vi "copyFuncArgAndNoteFromIniToTable.vi"(8 "valInCol5":string, 9 "valInCol2":string, 10 "valInCol1":string, 11 "arrayAtTheSameRow":string[](array[string])) -> (3 "arrWithFunc&Arg&Note":string[](array[string]))   [LabVIEW 2010]
panel:
  # "func"
  # "arg"
  # "note"
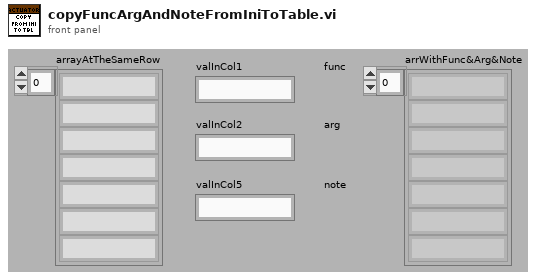
[diagram p1: front panel]
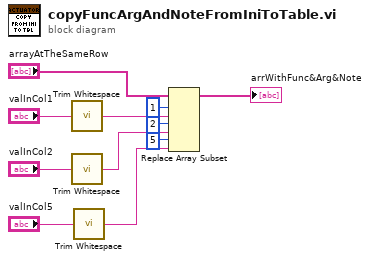
[diagram p0: block diagram]
diagram:
  n1 = call <vilib>:"Trim Whitespace.vi"("string"="valInCol1") -> ("trimmed string"=w5:string)  [unwired: 1 in]
  n2 = call <vilib>:"Trim Whitespace.vi"("string"="valInCol2") -> ("trimmed string"=w4:string)  [unwired: 1 in]
  n3 = call <vilib>:"Trim Whitespace.vi"("string"="valInCol5") -> ("trimmed string"=w3:string)  [unwired: 1 in]
  n4 = Replace Array Subset(array="arrayAtTheSameRow", new element #1=w5, index #1=1 ("index"), new element #2=w4, index #2=2 ("index"), new element #3=w3, index #3=5 ("index")) -> (→"arrWithFunc&Arg&Note":string[])
